vi "Parse LAMMPS .dat file.vi"(11 "Path":path) -> (2 "Structures Array":T1(array[cluster]), 3 "Timestamps":dbl[](array[numeric]))   [LabVIEW 2010]
panel:
  out "Array":string[][](array[string])
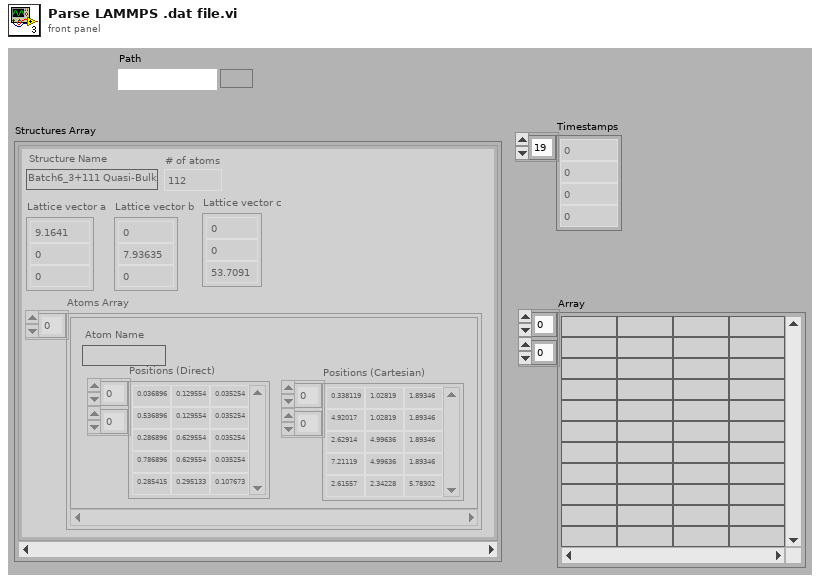
[diagram p1: front panel]
types:
  T1 = cluster{"Structure Name":string, "Lattice vector a":dbl[], "Lattice vector b":dbl[], "Lattice vector c":dbl[], "Atoms Array":cluster{"Atom Name":string, "Positions (Direct)":dbl[][], "Positions (Cartesian)":dbl[][]}[], "# of atoms":i32}[]
  T2 = cluster{"Atom Name":string, "Positions (Direct)":dbl[][], "Positions (Cartesian)":dbl[][]}[]
  T3 = cluster{"Input Array[0]":string, "Lattice vector c":dbl[][], dbl[][]}
  T4 = cluster{"Input Array[0]":string, "Lattice vector c":dbl[][], "Positions (Cartesian)":dbl[][]}[]
  T5 = cluster{"Atom Name":string, "Positions (Direct)":dbl[][], "Positions (Cartesian)":dbl[][]}
  T6 = cluster{"Atom Name":string, "Positions (Direct)":dbl[][], dbl[][]}
  T7 = cluster{string, "Lattice vector c":dbl[], "Lattice vector c":dbl[], "Lattice vector c":dbl[], cluster{"Atom Name":string, "Positions (Direct)":dbl[][], "Positions (Cartesian)":dbl[][]}[], i32}
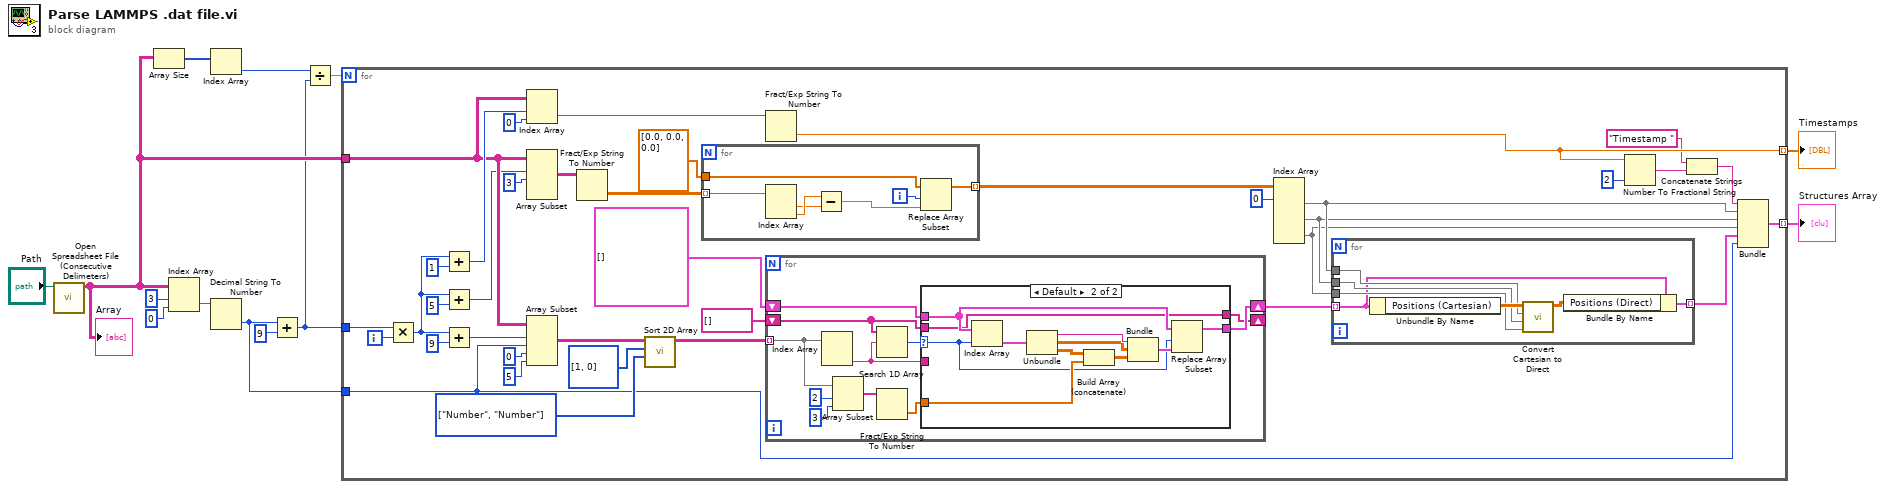
[diagram p0: block diagram]
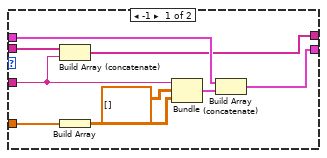
[diagram p2: hidden frame]
diagram:
  n1 = call "Open Spreadsheet File (Consecutive Delimeters).vi"("File"="Path") -> ("Array"=w9:string[][])  [unwired: 9 in, 1 out]
  "Array" <- w9
  n2 = Array Size(array=w9) -> (size(s)=w8:i32[])
  n3 = Index Array(array=w9, index (row)=3, index (col)=0 ("disabled index (col)")) -> (element=w10:string)
  n4 = Index Array(array=w8) -> (element=w7:i32)  [unwired: 1 in]
  n5 = Decimal String To Number(string=w10) -> (number=w3:i32)  [unwired: 2 in, 1 out]
  n6 = Add(x=w3, y=9) -> (x+y=w5:i32)
  n7 = Divide(x=w7, y=w5) -> (x/y=w4:dbl)
  n8 = for {
    N: w4 -> [_]
    tunnel: w9 -> [w28]
    tunnel: w5 -> [w48]
    tunnel: w3 -> [w35]
    tunnel: [w34] -> w1 mode=indexing
    tunnel: [w33] -> w2 mode=indexing
    i -> [w51]
    w39 = enum16{"String", "Number", "Date-Time"}[] [enum."Number", enum."Number"] items=["String", "Number", "Date-Time"] ("Sort by Datatype Array")
    n9 = Multiply(x=w48, y=w51) -> (x*y=w27:i32)
    n10 = Add(x=w27, y=1) -> (x+y=w44:i32)
    n11 = Add(x=w27, y=5) -> (x+y=w25:i32)
    n12 = Add(x=w27, y=9) -> (x+y=w47:i32)
    n13 = Index Array(array=w28, index (row)=w44, index (col)=0 ("disabled index (col)")) -> (element=w42:string)
    n14 = Array Subset(array=w28, index (row)=w25, length (row)=3 ("length")) -> (w23:string[][])  [unwired: 2 in]
    n15 = Array Subset(array=w28, index (row)=w47, length (row)=w35, index (col)=0 ("index"), length (col)=5 ("length")) -> (w41:string[][])
    n16 = Fract/Exp String To Number(string=w23) -> (number=w22:dbl[][])  [unwired: 3 in, 1 out]
    n17 = call "Sort 2D Array.vi"("Sort by Datatype Array"=w39, "Sort by Cols"=i32[] [1, 0], "Input Array"=w41) -> ("Output Array"=w38:string[][])  [unwired: 8 in]
    n18 = for {
      tunnel: w22 -> [w65] mode=indexing
      tunnel: dbl[] [0.0, 0.0, 0.0] ("Lattice vector c") -> [w62]
      tunnel: [w59] -> w20 mode=indexing
      i -> [w60]
      n19 = Index Array(array=w65) -> (element #1=w63:dbl, element #2=w64:dbl)  [unwired: 2 in]
      n20 = Subtract(x=w64, y=w63) -> (x-y=w61:dbl)
      n21 = Replace Array Subset(array=w62, new element=w61, index=w60) -> (w59:dbl[])
    }
    n22 = Fract/Exp String To Number(string=w42) -> (number=w34:dbl)  [unwired: 3 in, 1 out]
    n23 = for {
      tunnel: w38 -> [w73] mode=indexing
      shift-right: [w68] -> w18
      shift-left: T2 [] ("Atoms Array") -> [w71]
      shift-right: [w66] -> _
      shift-left: string[] [] -> [w67]
      n24 = Index Array(array=w73) -> (element #2=w70:string)  [unwired: 2 in, 1 out]
      n25 = Array Subset(array=w73, index=2, length=3) -> (w74:string[])
      n26 = Search 1D Array(1D array=w67, element=w70) -> (index of element=w72:i32)  [unwired: 1 in]
      n27 = Fract/Exp String To Number(string=w74) -> (number=w69:dbl[])  [unwired: 3 in, 1 out]
      n28 = case shown="Default" w72 {
        selector: w72 -> [_ w88]
        tunnel: w71 -> [w85 w90]
        tunnel: w70 -> [w78 _]
        tunnel: w69 -> [w84 w91]
        tunnel: [w83 w87] -> w68
        tunnel: w67 -> [w79 w86]
        tunnel: [w77 w86] -> w66
        frame -1 {
          n29 = Build Array (concatenate)(w79, w78) -> (w77:string[])
          n30 = Build Array(w84) -> (w82:dbl[][])
          n31 = Bundle("Input Array[0]"=w78, "Lattice vector c"=dbl[][] [], w82) -> (w80:T3)  [unwired: 1 in]
          n32 = Build Array (concatenate)(w85, w80) -> (w83:T4)
        }
        frame Default {
          n33 = Index Array(array=w90, index=w88) -> (element=w96:T5)
          n34 = Unbundle(w96) -> ("Atom Name"=w95:string, "Positions (Direct)"=w94:dbl[][], "Positions (Cartesian)"=w93:dbl[][])
          n35 = Build Array (concatenate)(w93, w91) -> (w92:dbl[][])
          n36 = Bundle("Atom Name"=w95, "Positions (Direct)"=w94, w92) -> (w89:T6)  [unwired: 1 in]
          n37 = Replace Array Subset(array=w90, new element=w89, index=w88) -> (w87:T2)
        }
      }
    }
    n38 = Index Array(array=w20, index (row) #1=0 ("index (row)")) -> (element #1=w17:dbl[], element #2=w16:dbl[], element #3=w15:dbl[])  [unwired: 5 in]
    n39 = for {
      tunnel: w18 -> [w54] mode=indexing
      tunnel: w17 -> [w57]
      tunnel: w16 -> [w56]
      tunnel: w15 -> [w55]
      tunnel: [w52] -> w14 mode=indexing
      n40 = Unbundle By Name(w54) -> ("Positions (Cartesian)"=w58:dbl[][])
      n41 = call "Convert Cartesian to Direct.vi"("Lattice vector c"=w55, "Lattice vector b"=w56, "Lattice vector a"=w57, "Positions (Cartesian)"=w58) -> ("Positions (Direct)"=w53:dbl[][])  [unwired: 7 in]
      n42 = Bundle By Name(cluster=w54, "Positions (Direct)"=w53) -> (w52:T5)
    }
    n43 = Number To Fractional String(number=w34, precision (6)=i16 2) -> (F-format string=w31:string)  [unwired: 2 in]
    n44 = Concatenate Strings("Timestamp " ("string"), w31) -> (w29:string)
    n45 = Bundle(w29, "Lattice vector c"=w17, "Lattice vector c"=w16, "Lattice vector c"=w15, w14, w35) -> (w33:T7)  [unwired: 1 in]
  }
  "Structures Array" <- w2
  "Timestamps" <- w1
